vi "MDAQ_MiniSum.vi"(10 "Status Cluster":T1 {"GATESTOP" format="%04x"; "GATESTRT" format="%04x"; "AMPLITUDE" format="%04x"; "M_CYCLES" format="%04x"; "N_CYCLES" format="%04x"; "STEP" format="%04x"; "BASE" format="%04x"; "CHAN" format="%04x"}, 11 "Spectrum":i32[](array[numeric])) -> (0 "sum":u32)   [LabVIEW 2021]
uses:
  HPGroup/MDAQ_LabVIEW/FunctionVIS/Status_Cluster.ctl
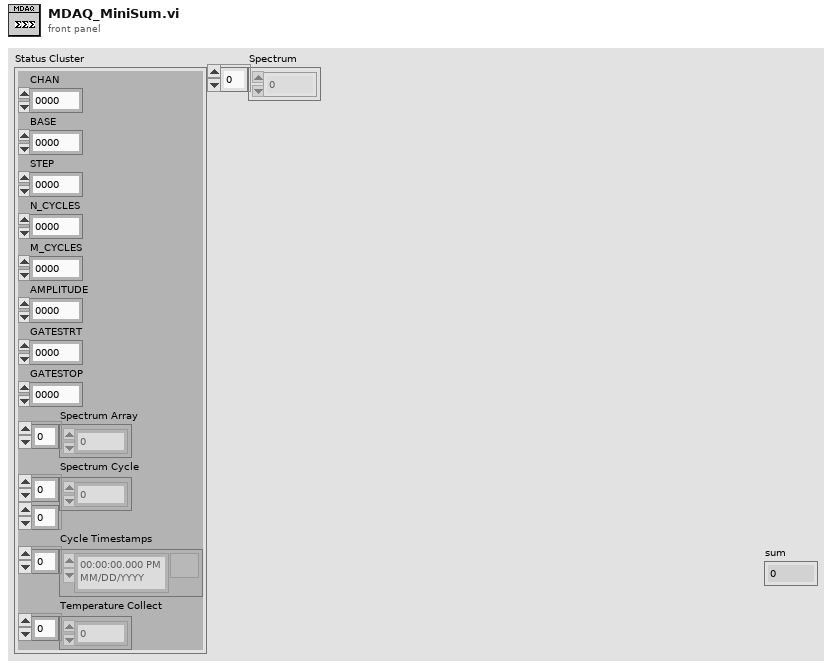
[diagram p1: front panel]
types:
  T1 = typedef "Status_Cluster.ctl" = cluster{"CHAN":u32, "BASE":u32, "STEP":u32, "N_CYCLES":u32, "M_CYCLES":u32, "AMPLITUDE":u32, "GATESTRT":u32, "GATESTOP":u32, "Spectrum Array":u32[], "Spectrum Cycle":u32[][], "Cycle Timestamps":timestamp[], "Temperature Collect":dbl[]}
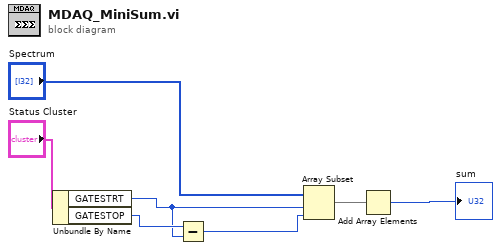
[diagram p0: block diagram]
diagram:
  n1 = Unbundle By Name("Status Cluster") -> ("GATESTRT"=w5:u32, "GATESTOP"=w6:u32)
  n2 = Subtract(x=w6, y=w5) -> (x-y=w4:u32)
  n3 = Array Subset(array="Spectrum", index=w5, length=w4) -> (w3:i32[])
  n4 = Add Array Elements(numeric array=w3) -> (sum=→"sum":i32)
